vi "magazine_open.vi"(8 "error in (no error)":errorcluster) -> (0 "error out":errorcluster)   [LabVIEW 2020]
uses:
  <vilib>/Rock Robotics/WPI/ThirdParty/Phoenix-LabVIEW/Motor Controller/Controls/CTRE_Phoenix_MotorControl_NeutralMode.ctl
  <vilib>/Rock Robotics/SystemInterfaces/DIO/FPGA_DIOChannel.ctl
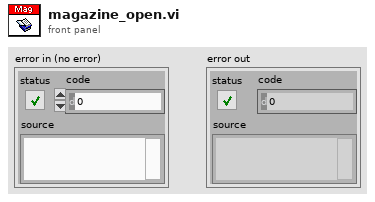
[diagram p1: front panel]
types:
  T1 = typedef "CTRE_Phoenix_MotorControl_NeutralMode.ctl" = enum8{"EEPROMSetting", "Override to Coast", "Override to Brake"}
  T2 = typedef "FPGA_DIOChannel.ctl" = enum8{"DIO 0", "DIO 1", "DIO 2", "DIO 3", "DIO 4", "DIO 5", "DIO 6", "DIO 7", "DIO 8", "DIO 9", "DIO MXP 0", "DIO MXP 1", "DIO MXP 2", "DIO MXP 3", "DIO MXP 4", "DIO MXP 5", "DIO MXP 6", "DIO MXP 7", "DIO MXP 8", "DIO MXP 9", "DIO MXP 10", "DIO MXP 11", "DIO MXP 12", "DIO MXP 13", "DIO MXP 14", "DIO MXP 15", "SPI Port CS1", "SPI Port CS2", "SPI Port CS3", "SPI Port MISO", "SPI Port MOSI", "Invalid"}
  T3 = typedef "WPI_MotorControlDeviceRef.ctl" = cluster{"DeviceStatus":errorcluster, "Type":T4, "PWM":cluster{"PWM Channel":T5, "DeadBand":T6}, "CAN":cluster{"Device Number":u8, "SetOutput VI Ref":variant, "GetOutput VI Ref":variant, "Enable VI Ref":variant, "Disable VI Ref":variant, "Data":variant}, "Invert":bool, "DIO PWM":cluster{"PWM \"Enable\" Channel":T5, "DIOChannel":T2, "PWM Rate":dbl}}
  T4 = typedef "WPI_MotorControlType.ctl" = enum16{"PWM", "CAN", "DIO PWM"}
  T5 = typedef "FPGA_DIOPWMChannel.ctl" = enum8{"PWM 0", "PWM 1", "PWM 2", "PWM 3", "PWM 4", "PWM 5", "PWM 6", "PWM 7", "PWM 8", "PWM 9", "PWM MXP 0", "PWM MXP 1", "PWM MXP 2", "PWM MXP 3", "PWM MXP 4", "PWM MXP 5", "PWM MXP 6", "PWM MXP 7", "PWM MXP 8", "PWM MXP 9", "Invalid"}
  T6 = typedef "WPI_PWMDeadband.ctl" = cluster{"Name":string, "maxPositivePwm":i32, "minPositivePwm":i32, "centerPwm":i32, "maxNegativePwm":i32, "minNegativePwm":i32, "angularRange":u16}
  T7 = typedef "WPI_DigitalInputDevRef.ctl" = cluster{"DevStatus":errorcluster, "DIO Channel":T2}
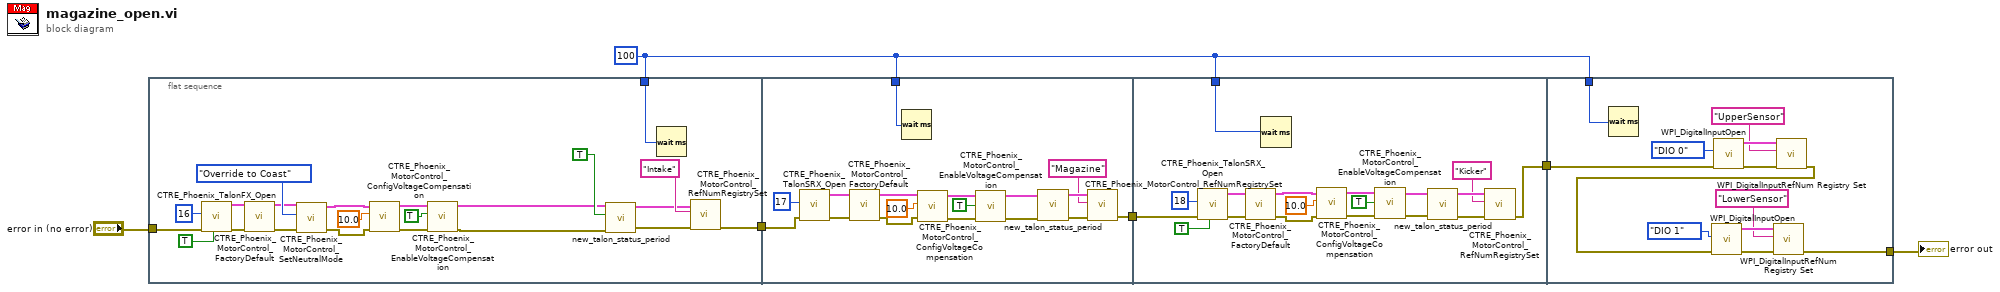
[diagram p0: block diagram]
diagram:
  w1 = u32 100 ("milliseconds to wait")
  n1 = flat-sequence {
    tunnel: "error in (no error)" -> [w28]
    tunnel: [w11] -> w2
    tunnel: w1 -> [w10]
    tunnel: [w31] -> w3
    tunnel: w2 -> [w30]
    tunnel: w1 -> [w29]
    tunnel: [w49] -> w4
    tunnel: w3 -> [w48]
    tunnel: w1 -> [w47]
    tunnel: [w66] -> w5
    tunnel: w4 -> [w65]
    tunnel: w1 -> [w64]
    frame #0 {
      n2 = call <vilib>:"CTRE_Phoenix_TalonFX_Open.vi"("Invert"=TRUE, "error in"=w28, "Device Number"=u8 16) -> ("error out"=w20:errorcluster, "PhoenixMotorControlDevRef"=w21:T3)  [unwired: 7 in]
      n3 = call <vilib>:"CTRE_Phoenix_MotorControl_FactoryDefault.vi"("error in"=w20, "PhoenixMotorControlDevRef"=w21) -> ("error out"=w25:errorcluster, "PhoenixMotorControlDevRef"=w24:T3)  [unwired: 8 in]
      n4 = call <vilib>:"CTRE_Phoenix_MotorControl_SetNeutralMode.vi"("error in (no error)"=w25, "Motor Control Neutral Mode"=CTRE_Phoenix_MotorControl_NeutralMode."Override to Coast", "PhoenixMotorControlDevRef"=w24) -> ("error out"=w14:errorcluster, "PhoenixMotorControlDevRef"=w15:T3)  [unwired: 7 in]
      n5 = call <vilib>:"CTRE_Phoenix_MotorControl_ConfigVoltageCompensation.vi"("error in (no error)"=w14, "Saturation Voltage"=10.0, "PhoenixMotorControlDevRef"=w15) -> ("error out"=w18:errorcluster, "PhoenixMotorControlDevRef"=w19:T3)  [unwired: 7 in]
      n6 = call <vilib>:"CTRE_Phoenix_MotorControl_EnableVoltageCompensation.vi"("error in (no error)"=w18, "Enable Voltage Compensation?"=TRUE, "PhoenixMotorControlDevRef"=w19) -> ("error out"=w7:errorcluster, "PhoenixMotorControlDevRef"=w8:T3)  [unwired: 7 in]
      n7 = call "new_talon_status_period.vi"("error in (no error)"=w7, "Feedback Data?"=TRUE, "PhoenixMotorControlDevRef"=w8) -> ("error out"=w12:errorcluster, "PhoenixMotorControlDevRef"=w13:T3)  [unwired: 7 in]
      n8 = Wait (ms)(milliseconds to wait=w10) -> ()  [unwired: 1 out]
      n9 = call <vilib>:"CTRE_Phoenix_MotorControl_RefNumRegistrySet.vi"("error in (no error)"=w12, "refnum name"="Intake", "PhoenixMotorControlDevRef"=w13) -> ("error out"=w11:errorcluster)  [unwired: 7 in, 1 out]
    }
    frame #1 {
      n10 = call <vilib>:"CTRE_Phoenix_TalonSRX_Open.vi"("error in"=w30, "Device Number"=u8 17) -> ("error out"=w36:errorcluster, "PhoenixMotorControlDevRef"=w41:T3)  [unwired: 8 in]
      n11 = call <vilib>:"CTRE_Phoenix_MotorControl_FactoryDefault.vi"("error in"=w36, "PhoenixMotorControlDevRef"=w41) -> ("error out"=w35:errorcluster, "PhoenixMotorControlDevRef"=w43:T3)  [unwired: 8 in]
      n12 = Wait (ms)(milliseconds to wait=w29) -> ()  [unwired: 1 out]
      n13 = call <vilib>:"CTRE_Phoenix_MotorControl_ConfigVoltageCompensation.vi"("error in (no error)"=w35, "Saturation Voltage"=10.0, "PhoenixMotorControlDevRef"=w43) -> ("error out"=w34:errorcluster, "PhoenixMotorControlDevRef"=w42:T3)  [unwired: 7 in]
      n14 = call <vilib>:"CTRE_Phoenix_MotorControl_EnableVoltageCompensation.vi"("error in (no error)"=w34, "Enable Voltage Compensation?"=TRUE, "PhoenixMotorControlDevRef"=w42) -> ("error out"=w33:errorcluster, "PhoenixMotorControlDevRef"=w44:T3)  [unwired: 7 in]
      n15 = call "new_talon_status_period.vi"("error in (no error)"=w33, "PhoenixMotorControlDevRef"=w44) -> ("error out"=w32:errorcluster, "PhoenixMotorControlDevRef"=w45:T3)  [unwired: 8 in]
      n16 = call <vilib>:"CTRE_Phoenix_MotorControl_RefNumRegistrySet.vi"("error in (no error)"=w32, "refnum name"="Magazine", "PhoenixMotorControlDevRef"=w45) -> ("error out"=w31:errorcluster)  [unwired: 7 in, 1 out]
    }
    frame #2 {
      n17 = call <vilib>:"CTRE_Phoenix_TalonSRX_Open.vi"("Invert"=TRUE, "error in"=w48, "Device Number"=u8 18) -> ("error out"=w55:errorcluster, "PhoenixMotorControlDevRef"=w54:T3)  [unwired: 7 in]
      n18 = call <vilib>:"CTRE_Phoenix_MotorControl_FactoryDefault.vi"("error in"=w55, "PhoenixMotorControlDevRef"=w54) -> ("error out"=w63:errorcluster, "PhoenixMotorControlDevRef"=w62:T3)  [unwired: 8 in]
      n19 = Wait (ms)(milliseconds to wait=w47) -> ()  [unwired: 1 out]
      n20 = call <vilib>:"CTRE_Phoenix_MotorControl_ConfigVoltageCompensation.vi"("error in (no error)"=w63, "Saturation Voltage"=10.0, "PhoenixMotorControlDevRef"=w62) -> ("error out"=w57:errorcluster, "PhoenixMotorControlDevRef"=w56:T3)  [unwired: 7 in]
      n21 = call <vilib>:"CTRE_Phoenix_MotorControl_EnableVoltageCompensation.vi"("error in (no error)"=w57, "Enable Voltage Compensation?"=TRUE, "PhoenixMotorControlDevRef"=w56) -> ("error out"=w59:errorcluster, "PhoenixMotorControlDevRef"=w58:T3)  [unwired: 7 in]
      n22 = call "new_talon_status_period.vi"("error in (no error)"=w59, "PhoenixMotorControlDevRef"=w58) -> ("error out"=w61:errorcluster, "PhoenixMotorControlDevRef"=w60:T3)  [unwired: 8 in]
      n23 = call <vilib>:"CTRE_Phoenix_MotorControl_RefNumRegistrySet.vi"("error in (no error)"=w61, "refnum name"="Kicker", "PhoenixMotorControlDevRef"=w60) -> ("error out"=w49:errorcluster)  [unwired: 7 in, 1 out]
    }
    frame #3 {
      n24 = Wait (ms)(milliseconds to wait=w64) -> ()  [unwired: 1 out]
      n25 = call <vilib>:"WPI_DigitalInputOpen.vi"("error in (no error)"=w65, "DIO Channel"=FPGA_DIOChannel."DIO 0") -> ("error out"=w74:errorcluster, "DigitalInputDevRef"=w73:T7)  [unwired: 8 in]
      n26 = call <vilib>:"WPI_DigitalInputRefNum Registry Set.vi"("error in (no error)"=w74, "refnum name"="UpperSensor", "DigitalInputDevRef"=w73) -> ("error out"=w75:errorcluster)  [unwired: 7 in, 1 out]
      n27 = call <vilib>:"WPI_DigitalInputOpen.vi"("error in (no error)"=w75, "DIO Channel"=FPGA_DIOChannel."DIO 1") -> ("error out"=w72:errorcluster, "DigitalInputDevRef"=w71:T7)  [unwired: 8 in]
      n28 = call <vilib>:"WPI_DigitalInputRefNum Registry Set.vi"("error in (no error)"=w72, "refnum name"="LowerSensor", "DigitalInputDevRef"=w71) -> ("error out"=w66:errorcluster)  [unwired: 7 in, 1 out]
    }
  }
  "error out" <- w5
